vi "LCB Log.vi"(8 "error in (no error)":errorcluster caption="Fehler (Eingang, kein Fehler)", 11 "Log Message":string) -> (0 "error out":errorcluster caption="Fehler (Ausgang)")   [LabVIEW 2021, in "labbCAN_Bus_API.lvlib"]
doc: "LCB_Func long __stdcall LCB_Log(const char *pLogMsg);"
uses:
  labbCAN_Bus_API.lvlib
  labbCAN_Bus_API.dll
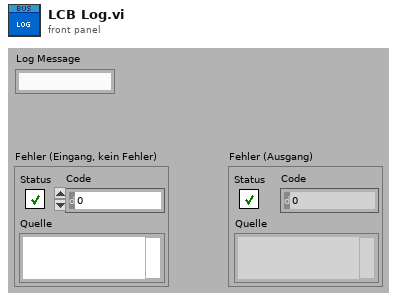
[diagram p1: front panel]
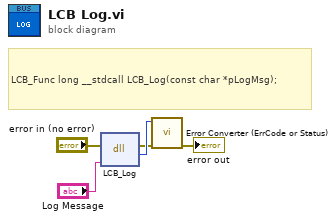
[diagram p0: block diagram]
diagram:
  # "LCB_Func long __stdcall LCB_Log(const char *pLogMsg);"
  n1 = dll-call lib="C:/Users/olaja/AppData/Local/CETONI_SDK/labbCAN_Bus_API.*" fn="LCB_Log"(error in="error in (no error)", "pLogMsg"="Log Message") -> (error out=w2:errorcluster, w3:i32)  [unwired: 3 in, 1 out]
  n2 = call "Error Converter (ErrCode or Status).vi"("error in (no error)"=w2, "error code"=w3) -> ("error out"=→"error out":errorcluster)  [unwired: 9 in]
